vi "Configuration Globals.vi"() -> ()   [LabVIEW 2017]
panel:
  in  "RT-host receiving port":u16
  in  "RT-host sending port":u16
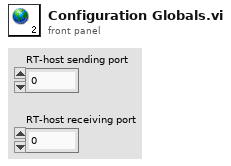
[diagram p1: front panel]
diagram:
